vi "PUMP RAMP 4 (SubVI).vi"(0 "Dynamic Data":dynamicdata(waveform), 1 "Numeric":i16, 2 "PUMP SELECTION":enum32{"PAM", "REGLO DIGITAL", "REGLO ANALOG"}(radio), 3 "Seq in":dbl[][](array[numeric])=[[20.0, 60.0, 40.0], [60.0, 40.0, 20.0], [100.0, 100.0, 100.0]], 9 "PORT (REGLO DIGITAL)":i32=7) -> (6 "to PAM input":bool[](array[boolean]), 7 "Rate (g/s)":dbl, 8 "to REGLO ANALOG":dbl, 10 "Weight (S1)":dbl, 11 "Step 2":i32, 12 "target reached":i32, 13 "x/y":dbl, 14 "Time (s)":dbl, 15 "bal_previous":i32, 17 "Target (g)":dbl, 18 "Waveform Chart 2":dynamicdata(graph))   [LabVIEW 2015]
uses:
  BERTTA.dll
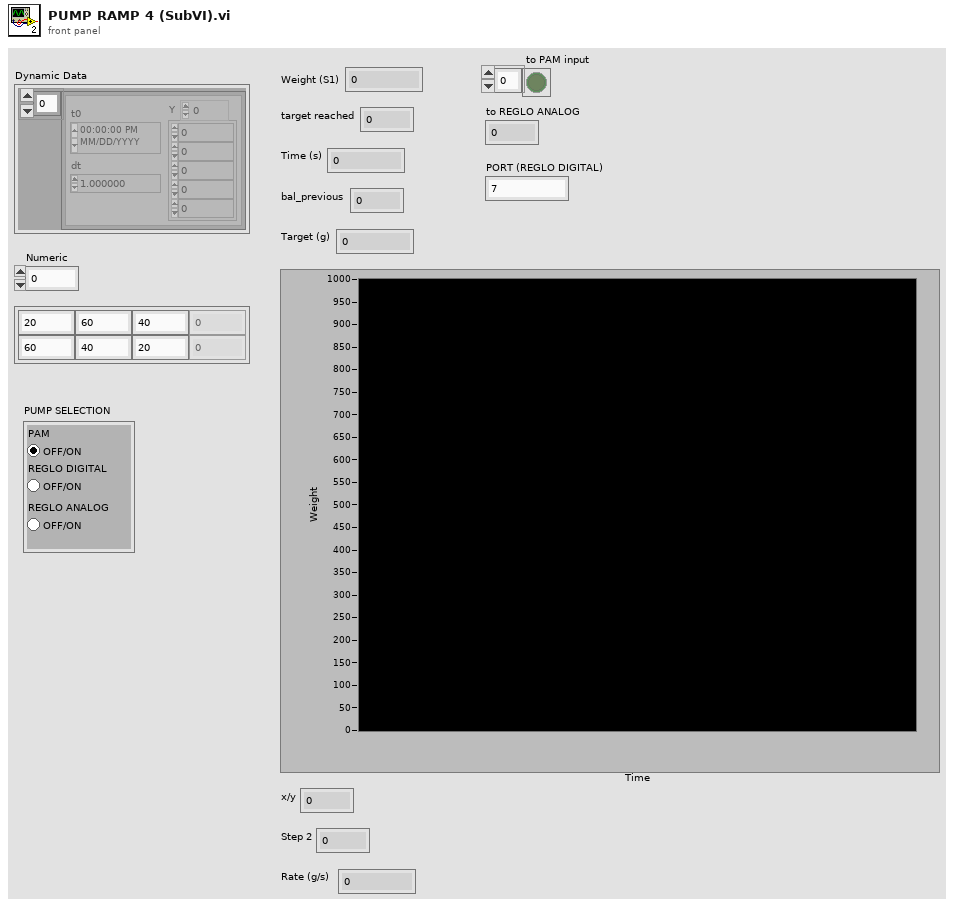
[diagram p1: front panel]
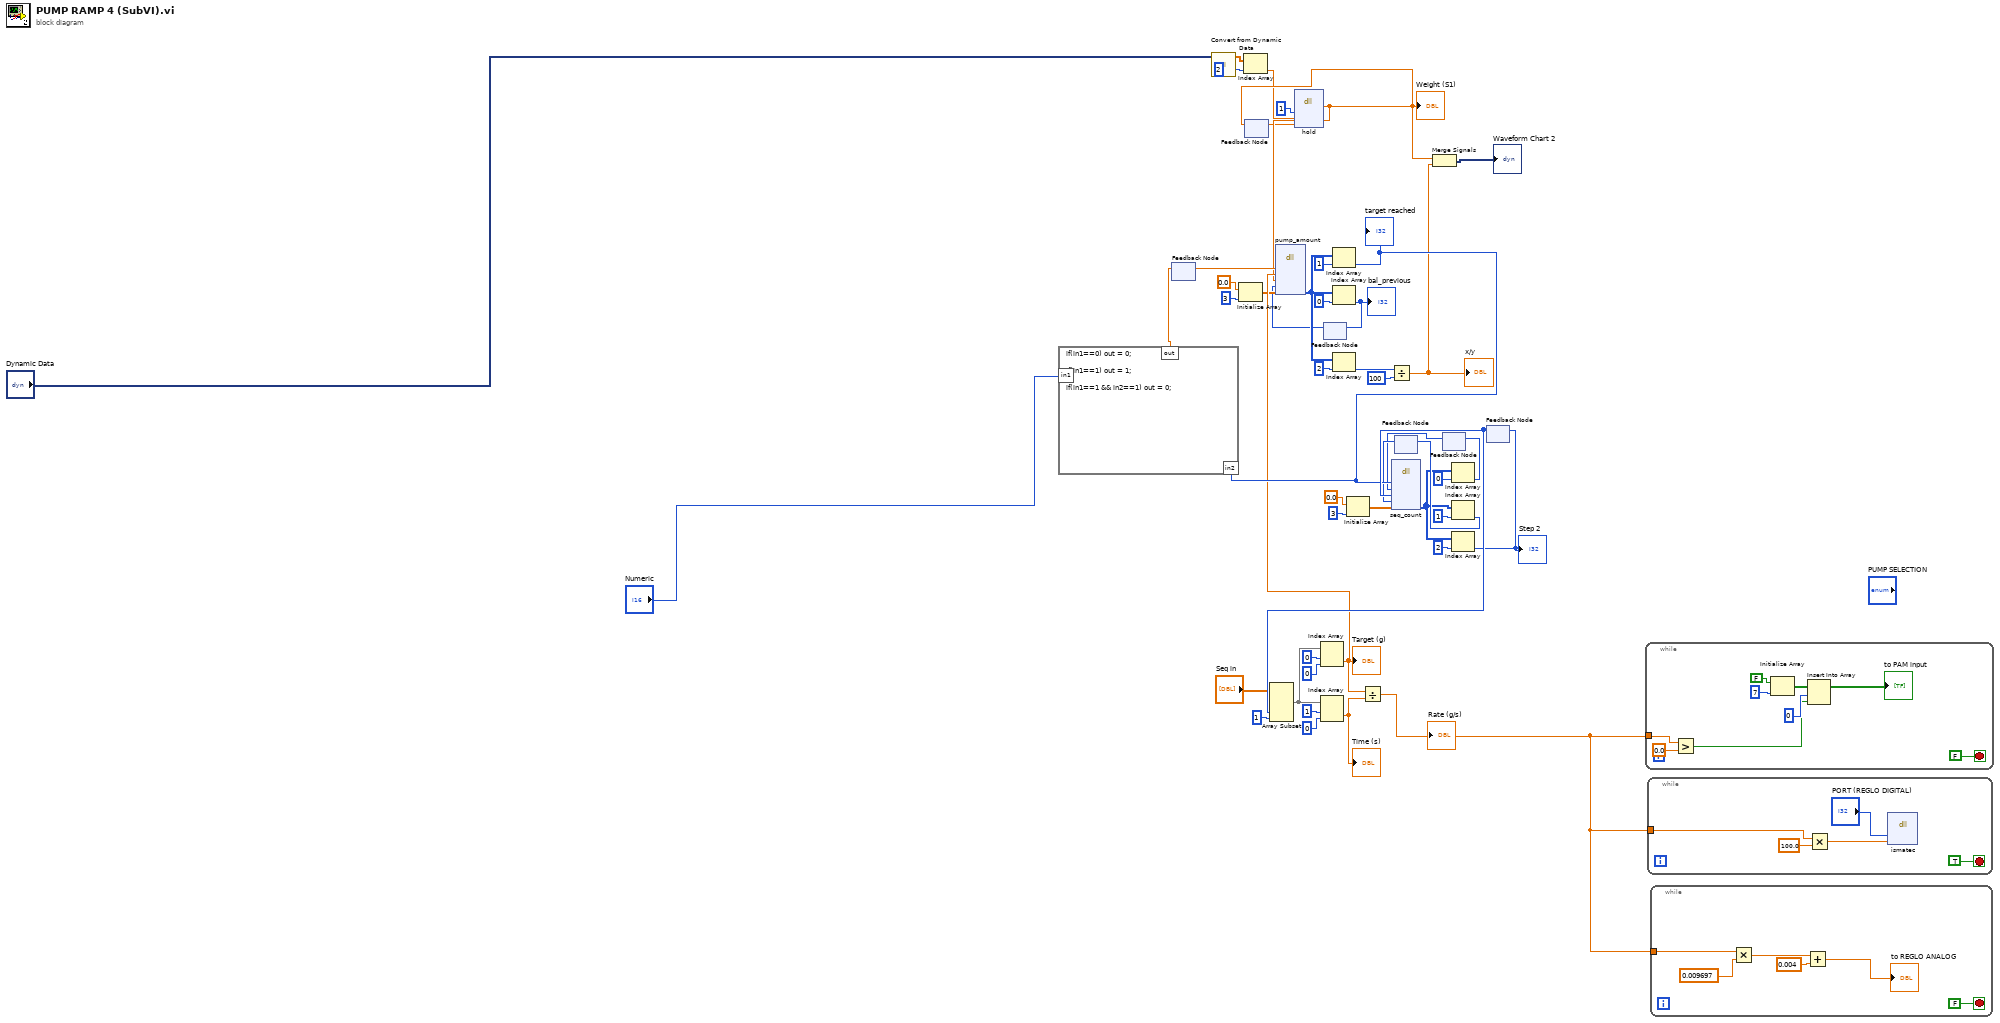
[diagram p0: block diagram]
diagram:
  n1 = feedback #1() -> (w44:dbl)  [unwired: 1 in]
  n2 = call "Convert from Dynamic Data"("Dynamic Data Type"="Dynamic Data") -> ("Array"=w11:dbl[])  [unwired: 3 in]
  n3 = Initialize Array(0.0 ("element"), 3 ("dimension size")) -> (w21:dbl[])
  n4 = Index Array(array=w11, index=2) -> (element=w12:dbl)
  n5 = feedback #2() -> (w13:dbl)  [unwired: 1 in]
  n6 = dll-call lib="C:/Users/xlaraser/Documents/Visual Studio 2017/Projects/Bertta/BERTTA/Debug/BERTTA.dll" fn="hold"("enable"=1, "in1"=w12, "in2"=w13) -> ("return type"=w24:dbl)  [unwired: 6 in, 2 out]
  "Weight (S1)" <- w24
  n7 = feedback-in #2(w24) -> ()
  n8 = feedback #3() -> (w18:i32)  [unwired: 1 in]
  n9 = Initialize Array(0.0 ("element"), 3 ("dimension size")) -> (w30:dbl[])
  n10 = feedback #4() -> (w38:i32)  [unwired: 1 in]
  n11 = feedback #5() -> (w37:i32)  [unwired: 1 in]
  n12 = feedback #6() -> (w46:i32)  [unwired: 1 in]
  n13 = Array Subset(array="Seq in", index (col)=w46, length (col)=1 ("length")) -> (w5:dbl[][])  [unwired: 2 in]
  n14 = Index Array(array=w5, index (row)=0, index (col)=0 ("disabled index (col)")) -> (element=w26:dbl)
  "Target (g)" <- w26
  n15 = dll-call lib="C:/Users/xlaraser/Documents/Visual Studio 2017/Projects/Bertta/BERTTA/Debug/BERTTA.dll" fn="pump_amount"("enable"=w44, "target"=w26, "bal"=w24, "bal_previous"=w18, "params"=w21) -> ("params"=w23:i32[])  [unwired: 8 in, 2 out]
  n16 = Index Array(array=w5, index (row)=1, index (col)=0 ("disabled index (col)")) -> (element=w9:dbl)
  "Time (s)" <- w9
  n17 = Index Array(array=w23, index=1) -> (element=w42:i32)
  "target reached" <- w42
  n18 = formula code="if(in1==0) out = 0;\n\nif(in1==1) out = 1;\n\nif(in1==1 && in2==1) out = 0;"("in1"="Numeric", "in2"=w42) -> ("out"=w43:dbl)
  n19 = feedback-in #1(w43) -> ()
  n20 = Index Array(array=w23, index=0) -> (element=w17:i32)
  "bal_previous" <- w17
  n21 = feedback-in #3(w17) -> ()
  n22 = Index Array(array=w23, index=2) -> (element=w27:i32)
  n23 = Divide(x=w26, y=w9) -> (x/y=w1:dbl)
  "Rate (g/s)" <- w1
  n24 = Divide(x=w27, y=100) -> (x/y=w28:dbl)
  "x/y" <- w28
  n25 = dll-call lib="C:/Users/xlaraser/Documents/Visual Studio 2017/Projects/Bertta/BERTTA/Debug/BERTTA.dll" fn="seq_count"("in1"=w42, "in2"=w37, "in3"=w46, "in4"=w38, "params"=w30) -> ("params"=w36:i32[])  [unwired: 8 in, 2 out]
  n26 = Merge Signals(w24, w28) -> (→"Waveform Chart 2":dynamicdata)
  n27 = Index Array(array=w36, index=0) -> (element=w39:i32)
  n28 = feedback-in #5(w39) -> ()
  n29 = Index Array(array=w36, index=1) -> (element=w40:i32)
  n30 = feedback-in #4(w40) -> ()
  n31 = Index Array(array=w36, index=2) -> (element=w45:i32)
  "Step 2" <- w45
  n32 = feedback-in #6(w45) -> ()
  n33 = while {
    tunnel: w1 -> [w49]
    stop <- FALSE stop-if-true
    n34 = Greater?(x=w49, y=0.0) -> (0:w50:bool)
    n35 = Initialize Array(FALSE ("element"), 7 ("dimension size")) -> (w54:bool[])
    n36 = Insert Into Array(array=w54, index=0, new element=w50) -> (→"to PAM input":bool[])
  }
  n37 = while {
    tunnel: w1 -> [w58]
    stop <- TRUE stop-if-true
    n38 = Multiply(x=w58, y=100.0) -> (x*y=w60:dbl)
    n39 = dll-call lib="C:/Users/xlaraser/Documents/Visual Studio 2017/Projects/Bertta/BERTTA/Debug/BERTTA.dll" fn="ismatec"("port"="PORT (REGLO DIGITAL)", "speed"=w60) -> ()  [unwired: 6 in, 2 out]
  }
  n40 = while {
    tunnel: w1 -> [w63]
    stop <- FALSE stop-if-true
    n41 = Multiply(x=w63, y=0.009697) -> (x*y=w65:dbl)
    n42 = Add(x=w65, y=0.004) -> (x+y=→"to REGLO ANALOG":dbl)
  }
